vi "Blueprint Editor UI.vi"(11 "Blueprint in":refnum<class "Blueprint.lvclass">) -> (3 "Blueprint":refnum<class "Blueprint.lvclass">)   [LabVIEW 2020, in "App.lvclass"]
uses:
  App.lvclass
  Blueprint/Blueprint.lvclass
  Item/Ingredient.ctl
  Item/Item.lvclass
  BP Item/BP Item.lvclass
  C:/Program Files (x86)/National Instruments/LabVIEW 2020/vi.lib/IlluminatedG/IG OOPanel/OOPanel/ArrayPanel/ArrayPanel.lvclass
  <vilib>/IlluminatedG/IG OOPanel/OOPanel/ArrayManager/ArrayManager.lvclass
panel:
  in  "Close":bool
  in  "Crafted At":string(combo)
  in  "Product Name":string
  in  "Craft Time":dbl
  in  "New Button":bool
  in  "Add Button":bool
  # "Components"
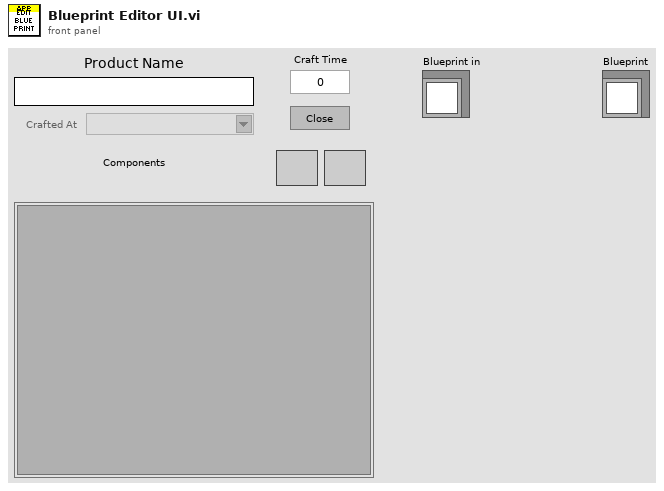
[diagram p1: front panel]
types:
  T1 = typedef "Item.lvclass/Ingredient.ctl" = cluster{"Item":refnum<class "Item.lvclass">, "Qty":dbl}
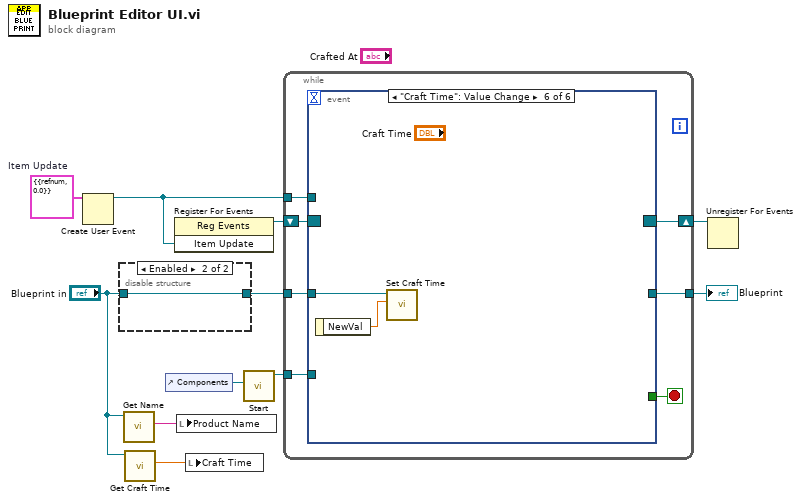
[diagram p0: block diagram]
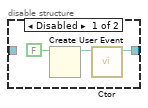
[diagram p2: hidden frame]
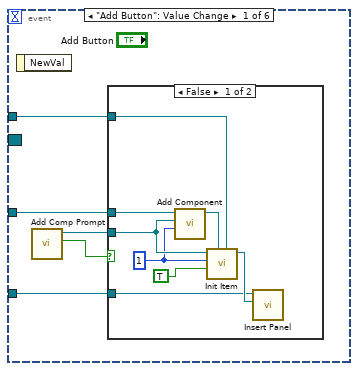
[diagram p3: hidden frame]
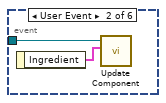
[diagram p5: hidden frame]
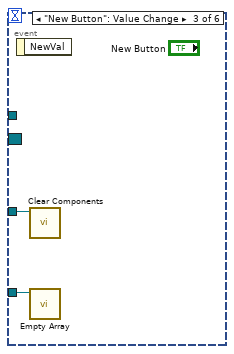
[diagram p6: hidden frame]
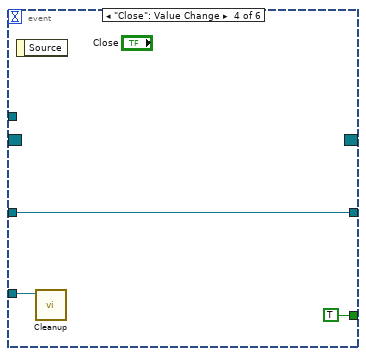
[diagram p7: hidden frame]
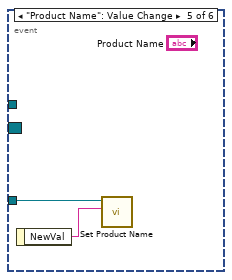
[diagram p8: hidden frame]
diagram:
  w5 = cluster{"Ingredient":T1} {"Ingredient"={"Item"=refnum, "Qty"=0.0}}  # Item Update
  n1 = Create User Event(user event datatype=w5) -> (user event=w8:refnum<user-event>)  [unwired: 1 in, 1 out]
  n2 = disable-structure shown="Enabled" {
    disable-tunnel: "Blueprint in" -> [_ w15]
    disable-tunnel: [w14 w15] -> w4
    frame Disabled {
      n3 = Create User Event(user event datatype=FALSE ("event data")) -> (user event=w12:refnum<user-event>)  [unwired: 1 in, 1 out]
      n4 = call "Ctor.vi"("Update Event"=w12) -> ("Blueprint out"=w14:refnum<class "Blueprint.lvclass">)  [unwired: 9 in, 1 out]
    }
    frame Enabled {
    }
  }
  n5 = call-dynamic "Get Name.vi"("Blueprint in"="Blueprint in") -> ("Name"=w3:string)  [unwired: 8 in, 2 out]
  n6 = call "Get Craft Time.vi"("Blueprint in"="Blueprint in") -> ("Craft Time"=w1:dbl)  [unwired: 8 in, 2 out]
  n7 = control-ref of="Components"() -> (w11:refnum<vi>)
  n8 = register-events(w8) -> (reference out=w7:refnum<event-registration>)  [unwired: 2 in, 1 out]
  n9 = local write "Product Name"(w3) -> ()
  n10 = local write "Craft Time"(w1) -> ()
  n11 = call <vilib>:"Start.vi"("Container"=w11) -> ("ArrayManager out"=w10:refnum<class "ArrayManager.lvclass">)  [unwired: 9 in, 1 out]
  n12 = while {
    tunnel: w10 -> [w22]
    tunnel: w4 -> [w21]
    tunnel: [w19] -> w9
    tunnel: w8 -> [w18]
    shift-right: [w16] -> w6
    shift-left: w7 -> [w17]
    stop <- w20 stop-if-true
    n13 = event shown="[5] \"Craft Time\": Value Change" {
      selector: w17 -> [_ _ _ _ _ _]
      dyn-events: [_ _ _ _ _ _] -> w16
      timeout: _ -> [_ _ _ _ _ _]
      tunnel: w22 -> [w25 _ w39 w40 _ _]
      tunnel: w21 -> [w24 w37 w38 w41 w44 w46]
      tunnel: [_ _ _ TRUE _ _] -> w20
      tunnel: [_ _ _ w41 _ _] -> w19
      tunnel: w18 -> [w23 _ _ _ _ _]
      event "Add Button": Value Change {
        n14 = event-data() -> ()  [unwired: 1 in, 1 out]
        n15 = call "Add Comp Prompt.vi"() -> ("Cancelled"=w26:bool, "Selected Component"=w27:refnum<class "Item.lvclass">)  [unwired: 10 in]
        n16 = case shown="False" w26 {
          tunnel: w27 -> [w33 _]
          tunnel: w25 -> [w28 _]
          tunnel: w24 -> [w35 _]
          tunnel: w23 -> [w30 _]
          frame False {
            w31 = 1 ("Qty")
            n17 = call "Add Component.vi"("Qty"=w31, "Item"=w33, "Blueprint in"=w35) -> ("Blueprint out"=w32:refnum<class "Blueprint.lvclass">)  [unwired: 7 in, 1 out]
            n18 = call "Init Item.vi"("Item Update"=w30, "Blueprint"=w32, "Removable? (F)"=TRUE ("Removable?"), "Qty"=w31, "Item"=w33) -> ("BP Item out"=w29:refnum<class "BP Item.lvclass">)  [unwired: 5 in, 1 out]
            n19 = call <vilib>:"Insert Panel.vi"("Panel/Type"=w29, "PanelArray in"=w28) -> ()  [unwired: 7 in, 3 out]
          }
          frame True {
          }
        }
      }
      event User Event {
        n20 = event-data() -> ("Ingredient"=w36:T1)  [unwired: 1 in]
        n21 = call "Update Component.vi"("Component"=w36, "Blueprint in"=w37) -> ()  [unwired: 8 in, 2 out]
      }
      event "New Button": Value Change {
        n22 = event-data() -> ()  [unwired: 1 in, 1 out]
        n23 = call "Clear Components.vi"("Blueprint in"=w38) -> ()  [unwired: 9 in, 2 out]
        n24 = call <vilib>:"Empty Array.vi"("ArrayManager in"=w39) -> ()  [unwired: 9 in, 2 out]
      }
      event "Close": Value Change {
        n25 = event-data() -> ()  [unwired: 1 in, 1 out]
        n26 = call <vilib>:"Cleanup.vi"("PanelArray in"=w40) -> ()  [unwired: 10 in, 1 out]
      }
      event "Product Name": Value Change {
        n27 = event-data() -> ("NewVal"=w43:string)  [unwired: 1 in]
        n28 = call "Set Product Name.vi"("Product Name"=w43, "Blueprint in"=w44) -> ()  [unwired: 8 in, 2 out]
      }
      event "Craft Time": Value Change {
        n29 = event-data() -> ("NewVal"=w45:dbl)  [unwired: 1 in]
        n30 = call "Set Craft Time.vi"("Craft Time"=w45, "Blueprint in"=w46) -> ()  [unwired: 8 in, 2 out]
      }
    }
  }
  "Blueprint" <- w9
  n31 = Unregister For Events(event registration refnum=w6) -> ()  [unwired: 1 in, 1 out]
